vi "UDT_loggingModule_formatFileData.vi"() -> (3 "Unit Test Framework Results":T1)   [LabVIEW 2017]
doc: "Use this template to create a user-defined test VI. Define your test requirements and wire the results to the <b>Result (Test)</b> control. Do not modify the <b>Unit Test Framework Results</b> indicator."
uses:
  <vilib>/utf/common/utf_test_result_troll.ctl
  <vilib>/utf/common/utf_test_result.ctl
  <vilib>/utf/common/utf_test_result_failure.ctl
  <vilib>/utf/common/utf_test_comparison_operators.ctl
  <vilib>/utf/common/utf_vi_tag.ctl
  RT/loggingModule/Queue/TypeDefs/queueFGVState.ctl
  RT/ErrorMonitor/Queue/TypeDefs/message.ctl
  RT/loggingModule/loggingModule.lvlib
  RT/ErrorMonitor/ErrorMonitor.lvlib
  <vilib>/Control Software Solutions Ltd/UTF Helper/Unit Test Helper.lvlib
  <vilib>/utf/NI_UnitTestFramework.lvlib
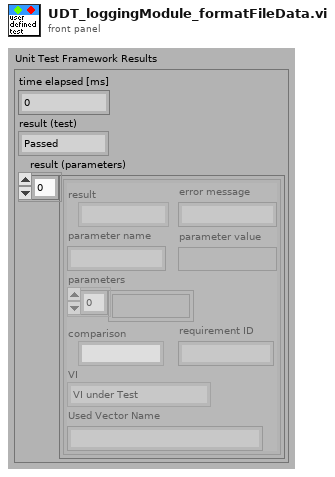
[diagram p1: front panel]
types:
  T1 = typedef "NI_UnitTestFramework.lvlib/utf_test_result_troll.ctl" = cluster{"time elapsed [ms]":u32, "result (test)":T2, "result (parameters)":T3[]}
  T2 = typedef "NI_UnitTestFramework.lvlib/utf_test_result.ctl" = enum16{"Passed", "Failed", "Error", "Skipped", "Not Processed"}
  T3 = typedef "NI_UnitTestFramework.lvlib/utf_test_result_failure.ctl" = cluster{"result":T2, "error message":string, "parameter name":string, "parameter value":variant, "parameters":variant[], "comparison":T4, "requirement ID":string, "VI":T5, "Used Vector Name":string}
  T4 = typedef "NI_UnitTestFramework.lvlib/utf_test_comparison_operators.ctl" = enum16{"=", "!=", ">", ">=", "<", "<=", "range", "symmetric tolerance", "asymmetric tolerance", "string contains", "string not contain", "array size", "string length", "array range", "by element", "array range (limit array)", "user-defined", "array contains", "array not contain", "vector length", "= (elm)", "!= (elm)", "= (case insensitive)", "!= (case insensitive)"}
  T5 = typedef "NI_UnitTestFramework.lvlib/utf_vi_tag.ctl" = enum16{"Setup VI", "VI under Test", "Teardown VI"}
  T6 = typedef "loggingModule.lvlib/queueFGVState.ctl" = enum16{"obtain", "enqueue low priority", "enqueue high priority", "dequeue", "release"}
  T7 = typedef "ErrorMonitor.lvlib/message.ctl" = cluster{"calling module":string, "message":string, "Data":variant}
  T8 = typedef "loggingModule.lvlib/message.ctl" = cluster{"calling module":string, "message":string, "data":variant}
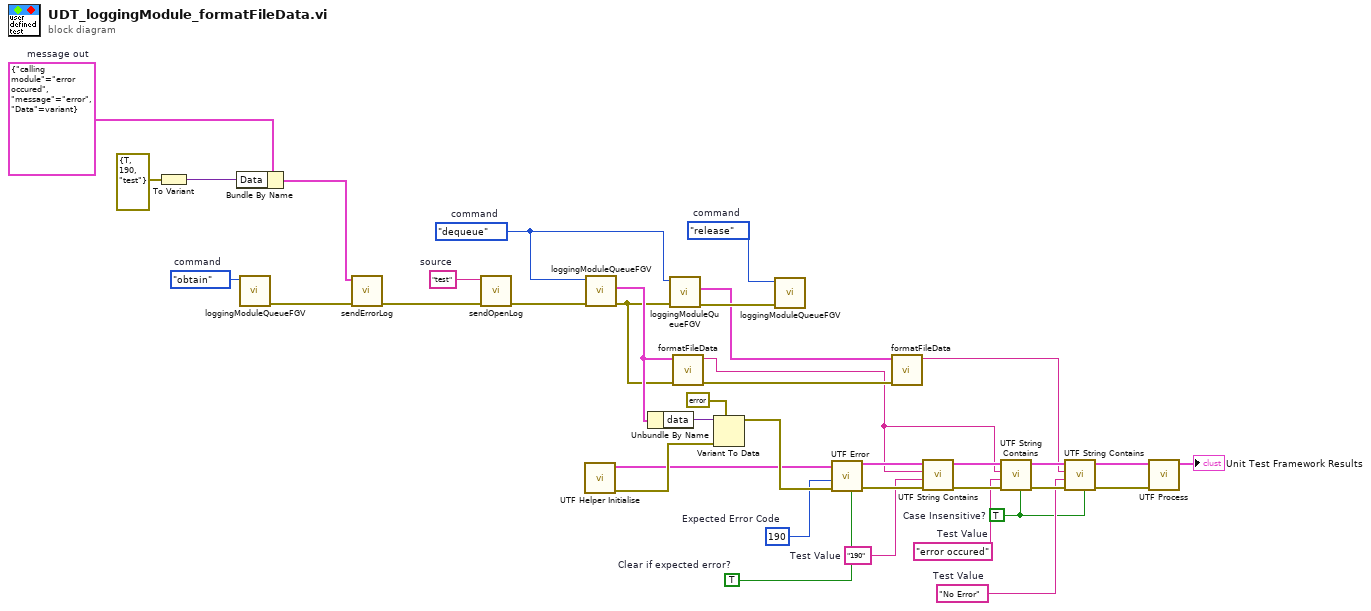
[diagram p0: block diagram]
diagram:
  w1 = TRUE  # Clear if expected error?
  w4 = TRUE  # Case Insensitive?
  w5 = "No Error"  # Test Value
  w9 = "error occured"  # Test Value
  w13 = "190"  # Test Value
  w18 = 190  # Expected Error Code
  w27 = queueFGVState."release"  # command
  w29 = queueFGVState."dequeue"  # command
  w33 = T7 {"calling module"="error occured", "message"="error", "Data"=variant}  # message out
  w35 = "test"  # source
  w38 = queueFGVState."obtain"  # command
  n1 = To Variant(anything=errorcluster {"status"=TRUE, "code"=190, "source"="test"} ("error constant")) -> (Variant=w32:variant)
  n2 = Bundle By Name(cluster=w33, "Data"=w32) -> (w31:T7)
  n3 = call "loggingModuleQueueFGV.vi"("command"=w38) -> ("error out"=w37:errorcluster)  [unwired: 9 in, 1 out]
  n4 = call "sendErrorLog.vi"("error in (no error)"=w37, "message out"=w31) -> ("error out"=w36:errorcluster)  [unwired: 9 in]
  n5 = call "sendOpenLog.vi"("error in (no error)"=w36, "source"=w35) -> ("error out"=w30:errorcluster)  [unwired: 9 in]
  n6 = call <vilib>:"UTF Helper Initialise.vi"() -> ("error out"=w21:errorcluster, "results array"=w19:T3[])  [unwired: 10 in]
  n7 = call "loggingModuleQueueFGV.vi"("error in (no error)"=w30, "command"=w29) -> ("error out"=w17:errorcluster, "message out"=w24:T8)  [unwired: 8 in]
  n8 = Unbundle By Name(w24) -> ("data"=w23:variant)
  n9 = call "loggingModuleQueueFGV.vi"("error in (no error)"=w17, "command"=w29) -> ("error out"=w28:errorcluster, "message out"=w25:T8)  [unwired: 8 in]
  n10 = call "formatFileData.vi"("error in (no error)"=w17, "message out"=w24) -> ("error out"=w16:errorcluster, "LogData"=w10:string)  [unwired: 8 in]
  n11 = Variant To Data(error in=w21, type=errorcluster {"status"=FALSE, "code"=0, "source"=""} ("error constant"), Variant=w23) -> (data=w20:errorcluster)  [unwired: 1 out]
  n12 = call "loggingModuleQueueFGV.vi"("error in (no error)"=w28, "command"=w27) -> ()  [unwired: 8 in, 2 out]
  n13 = call <vilib>:"UTF Error.vi"("Clear if expected error?"=w1, "error in (no error)"=w20, "Expected Error Code"=w18, "Input Results"=w19) -> ("error out"=w14:errorcluster, "Output Results"=w15:T3[])  [unwired: 6 in]
  n14 = call "formatFileData.vi"("error in (no error)"=w16, "message out"=w25) -> ("LogData"=w6:string)  [unwired: 8 in, 1 out]
  n15 = call <vilib>:"UTF String Contains.vi"("error in (no error)"=w14, "Test Value"=w13, "Input"=w10, "Input Results"=w15) -> ("error out"=w11:errorcluster, "Output Results"=w12:T3[])  [unwired: 6 in]
  n16 = call <vilib>:"UTF String Contains.vi"("Case Insensitive?"=w4, "error in (no error)"=w11, "Test Value"=w9, "Input"=w10, "Input Results"=w12) -> ("error out"=w7:errorcluster, "Output Results"=w8:T3[])  [unwired: 5 in]
  n17 = call <vilib>:"UTF String Contains.vi"("Case Insensitive?"=w4, "error in (no error)"=w7, "Test Value"=w5, "Input"=w6, "Input Results"=w8) -> ("error out"=w3:errorcluster, "Output Results"=w2:T3[])  [unwired: 5 in]
  n18 = call <vilib>:"UTF Process.vi"("error in (no error)"=w3, "results array"=w2) -> ("Unit Test Framework Results"=→"Unit Test Framework Results":T1)  [unwired: 9 in]
